vi "SVFA Power Spectral Density (1 Ch).vi"(0 "scaled signal [EU]":waveform(dbl), 2 "window":T8=1 items=["None"=0, "Hanning"=1, "Hamming"=2, "Blackman-Harris"=3, "Exact Blackman"=4, "Blackman"=5, "Flat Top"=6, "4 Term B-Harris "=7, "7 Term B-Harris"=8, "Low Sidelobe"=9, "Force"=64, "Exponential"=65, "Blackman Nuttall"=11, "Triangle"=30, "Bartlett-Hanning"=31, "Bohman"=32, "Parzen"=33, "Welch"=34, "Kaiser"=60, "Dolph-Chebyshev"=61, "Gaussian"=62], 4 "dB On (F)":bool, 5 "error in (no error)":errorcluster, 6 "desired units":enum16{"EU^2 / Hz", "EU / sqrt(Hz)"}(ring), 7 "averaging parameters":T7={"averaging mode"=enum."No averaging", "weighting mode"=enum."Exponential", "number of averages"=10, "linear mode"=enum."One shot"} {"number of averages" min=1 step=1}, 9 "restart averaging (F)":bool) -> (11 "averaging done":bool, 13 "averages completed":dbl, 14 "power spectral density [EU^2 rms / Hz]":cluster{"f0":dbl, "df":dbl, "magnitude":dbl[]}={"f0"=nan, "df"=inf, "magnitude"=[]} {"magnitude" format="%.2p"; "df" format="%.2p"; "f0" format="%.2p"}, 15 "unit label":string, 18 "spectrum info":T1={"channel name"="", "description"="", "x-axis units"=0, "spectral info"={"spectrum type"=enum."Power [Magnitude^2]", "linear/dB"=enum."linear", "window"=0, "window size"=0, "FFT size"=0}, "engineering units"=0, "custom label"="", "dB reference [EU]"=0.0, "peak units"=enum."rms", "weighting filter"=0, "spectral density?"=FALSE, "unit label"="", "spectrum skewed?"=FALSE, "complimentary spectrum units"=enum."none"} {"x-axis units" items=["Time (s)"=0, "Frequency-CB (Hz)"=1, "Frequency-CPB (Hz)"=1248, "Frequency-Arbitrary (Hz)"=2357, "Quefrency (s)"=2, "Revolutions (rev)"=3, "Order"=4, "Speed (RPM)"=11, "Speed (rad/s)"=21, "Index"=65535]; "weighting filter" items=["Linear", "A-weighting", "B-weighting", "C-weighting", "ITU-R 468-4", "Dolby", "CCITT", "C-message", "Wb", "Wc", "Wd", "We", "Wf", "Wh", "Wj", "Wk", "Wm", "AES17 20 kHz lowpass", "AES17 40 kHz lowpass", "AES17 20 kHz highpass", "AES17 40 kHz highpass"]; "dB reference [EU]" format="%.2f"; "engineering units" items=["custom..."=0, "V"=1, "A"=21, "C"=30, "pC"=31, "s"=32, "-"=29, "Pa"=2, "N"=20, "g"=3, "m/s^2"=4, "m/s"=5, "m"=6, "mm/s"=12, "mm"=13, "micron/s"=14, "micron"=15, "in/s^2"=7, "in/s"=8, "in"=9, "mil/s"=10, "mil"=11, "rad/s^2"=16, "rad/s"=17, "rad"=18, "deg/s^2"=26, "deg/s"=27, "deg"=28, "RPM"=22, "cycle/s^2"=23, "Hz"=24, "cycle"=25, "strain"=19]; "spectral info"."window" items=["None "=0, "Hanning"=1, "Hamming"=2, "Blackman-Harris"=3, "Exact Blackman"=4, "Blackman"=5, "Flat Top"=6, "4 Term B-Harris "=7, "7 Term B-Harris"=8, "Low Sidelobe"=9, "Force - Exponential"=10, "Gaussian"=62]}, 19 "error out":errorcluster)   [LabVIEW 2017]
doc: "Computes the power spectral density of <B>scaled signal [EU]</B> and returns the result in the selected units. Use the power spectral density to make repeatable measurements of the noise floor that are independent of the block size. Wire data to the <B>scaled signal [EU]</B> input to determine the polymorphic instance to use or manually select the instance."
uses:
  <vilib>/addons/_NISVFA/_Shared subVIs/Controls/svc_Window.ctl
  <vilib>/addons/_NISVFA/_Shared subVIs/Controls/svc_Spectrum Info.ctl
  <vilib>/addons/_NISVFA/_Shared subVIs/Controls/svc_X-Axis Units.ctl
  <vilib>/addons/_NISVFA/_Shared subVIs/Controls/svc_Spectrum Type.ctl
  <vilib>/addons/_NISVFA/_Shared subVIs/Controls/svc_Engineering Units Text Ring.ctl
  <vilib>/addons/_NISVFA/_Shared subVIs/Controls/svc_Weighting Filter Text Ring.ctl
  <vilib>/addons/_NISVFA/_Shared subVIs/Controls/svc_Complimentary Spectrum Units.ctl
  <vilib>/Analysis/2dsp.llb/Power Spectrum (DBL).vi
  <vilib>/Analysis/2dsp.llb/Real FFT.vi
  <vilib>/addons/_NISVFA/_Shared subVIs/Windowing/svfa_Scaled Time Domain Window (Array).vi
  <vilib>/addons/_NISVFA/_Shared subVIs/Common/svc_Get SV Channel Info.vi
  <vilib>/addons/_NISVFA/_Shared subVIs/Spectrum Averaging/svfa_No Average Array (complex).vi
  <vilib>/addons/_NISVFA/_Shared subVIs/Spectrum Averaging/svfa_Average Array (complex).vi
  <vilib>/addons/_NISVFA/_Spectrum Processing/subVIs/svfa_Peak to RMS to Peak2Peak.vi
  <vilib>/addons/_NISVFA/_Spectrum Processing/subVIs/svfa_Mag to Mag2.vi
  <vilib>/addons/_NISVFA/_Spectrum Processing/subVIs/svfa_Linear to dB.vi
  <vilib>/addons/_NISVFA/_Spectrum Processing/subVIs/svfa_dBrefA to dBrefB.vi
  <vilib>/addons/_NISVFA/_Spectrum Processing/subVIs/svfa_Spectrum to Spectral Density.vi
  <vilib>/Analysis/4window.llb/Force Window.vi
  <vilib>/Analysis/4window.llb/Force Window (DBL).vi
  <vilib>/Analysis/4window.llb/Exponential Window.vi
  <vilib>/Analysis/4window.llb/Exponential Window (DBL).vi
  <vilib>/addons/_NISVFA/_Shared subVIs/Common/svc_Get Weighting Enum and Labels.vi
  <vilib>/addons/_NISVFA/_Shared subVIs/Common/svc_Unit Label Lexical Class.vi
  <vilib>/addons/_NISVFA/_Shared subVIs/Common/svc_Engineering Units to Unit Label.vi
  <vilib>/addons/_NISVFA/_Shared subVIs/Common/svc_Format Value (DBL).vi
  <vilib>/addons/_NISVFA/_Shared subVIs/Common/svc_Window Parameters.vi
  <vilib>/Utility/error.llb/Error Cluster From Error Code.vi
  <vilib>/Analysis/0measdsp.llb/Scaled Time Domain Window.vi
  <vilib>/Analysis/0measdsp.llb/Scaled Time Domain Window (DBL).vi
  <vilib>/addons/_NISVFA/_Spectrum Processing/subVIs/svfa_Spectrum Info Window to windowTd Type Def.vi
  <vilib>/addons/_NISVFA/_Shared subVIs/Common/svc_Get Window Info.vi
  <vilib>/addons/_NISVFA/_Shared subVIs/Common/svc_Channel Info to Spectrum Info.vi
  <vilib>/addons/_NISVFA/_Shared subVIs/Common/svc_Unit Label to Engineering Units.vi
  <vilib>/Analysis/NI_AALPro.lvlib
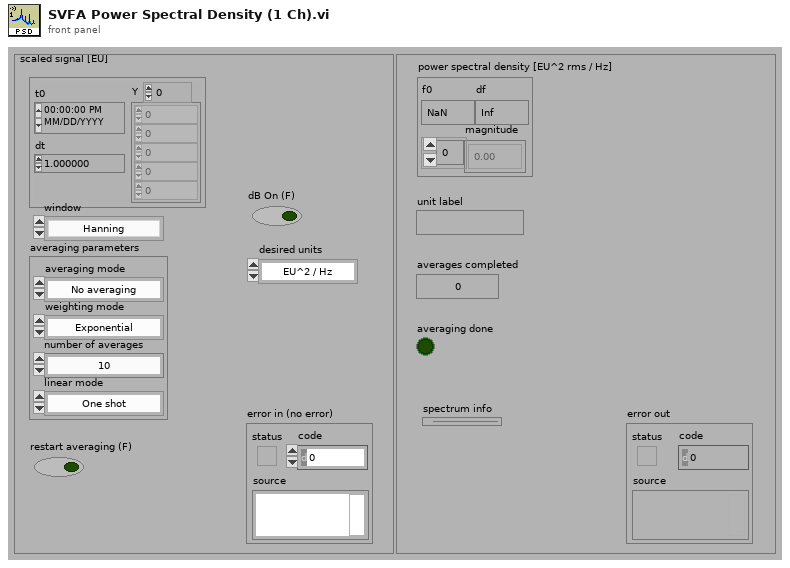
[diagram p1: front panel]
types:
  T1 = typedef "svc_Spectrum Info.ctl" = cluster{"channel name":string, "description":string, "x-axis units":T2, "spectral info":cluster{"spectrum type":T3, "linear/dB":enum16{"linear", "dB"}, "window":u16, "window size":i32, "FFT size":i32}, "engineering units":T4, "custom label":string, "dB reference [EU]":dbl, "peak units":enum16{"rms", "peak", "peak-peak"}, "weighting filter":T5, "spectral density?":bool, "unit label":string, "spectrum skewed?":bool, "complimentary spectrum units":T6}
  T2 = typedef "svc_X-Axis Units.ctl" = u16
  T3 = typedef "svc_Spectrum Type.ctl" = enum16{"FFT Spectrum [complex]", "Amplitude [Magnitude]", "Power [Magnitude^2]", "Cross Spectrum [complex]", "Frequency Response [Complex]"}
  T4 = typedef "svc_Engineering Units Text Ring.ctl" = u16
  T5 = typedef "svc_Weighting Filter Text Ring.ctl" = u16
  T6 = typedef "svc_Complimentary Spectrum Units.ctl" = enum16{"none", "radians", "degrees", "cycles", "imaginary"}
  T7 = cluster{"averaging mode":enum16{"No averaging", "Vector averaging", "RMS averaging", "Peak hold"}, "weighting mode":enum16{"Linear", "Exponential"}, "number of averages":u32, "linear mode":enum16{"One shot", "Auto restart"}}
  T8 = typedef "svc_Window.ctl" = u32
  T9 = cluster{"linear/dB":enum16{"no change", "linear", "dB"}, "dB reference (0: no change)":dbl, "power/magnitude":enum16{"no change", "power", "magnitude"}, "view":enum16{"no change", "rms", "peak", "peak-peak"}}
  T10 = enum16{"Restart processing", "Continue processing", "Skip processing"}
  T11 = enum16{"no change", "spectrum", "spectral density"}
  T12 = enum16{"No averaging", "Vector averaging", "RMS averaging", "Peak hold"}
  T13 = cluster{"complex FFT":cdb[], "real FFT":dbl[], "f0":dbl, "df":dbl, "averages completed":dbl, "averaging parameters":cluster{"averaging mode":enum16{"No averaging", "Vector averaging", "RMS averaging", "Peak hold"}, "weighting mode":enum16{"Linear", "Exponential"}, "number of averages":u32, "linear mode":enum16{"One shot", "Auto restart"}}}
  T14 = cluster{"complex FFT":cdb[], "Mag/Real FFT":dbl[], "f0":dbl, "df":dbl, "averages completed":dbl, "averaging parameters":cluster{"averaging mode":enum16{"No averaging", "Vector averaging", "RMS averaging", "Peak hold"}, "weighting mode":enum16{"Linear", "Exponential"}, "number of averages":u32, "linear mode":enum16{"One shot", "Auto restart"}}}
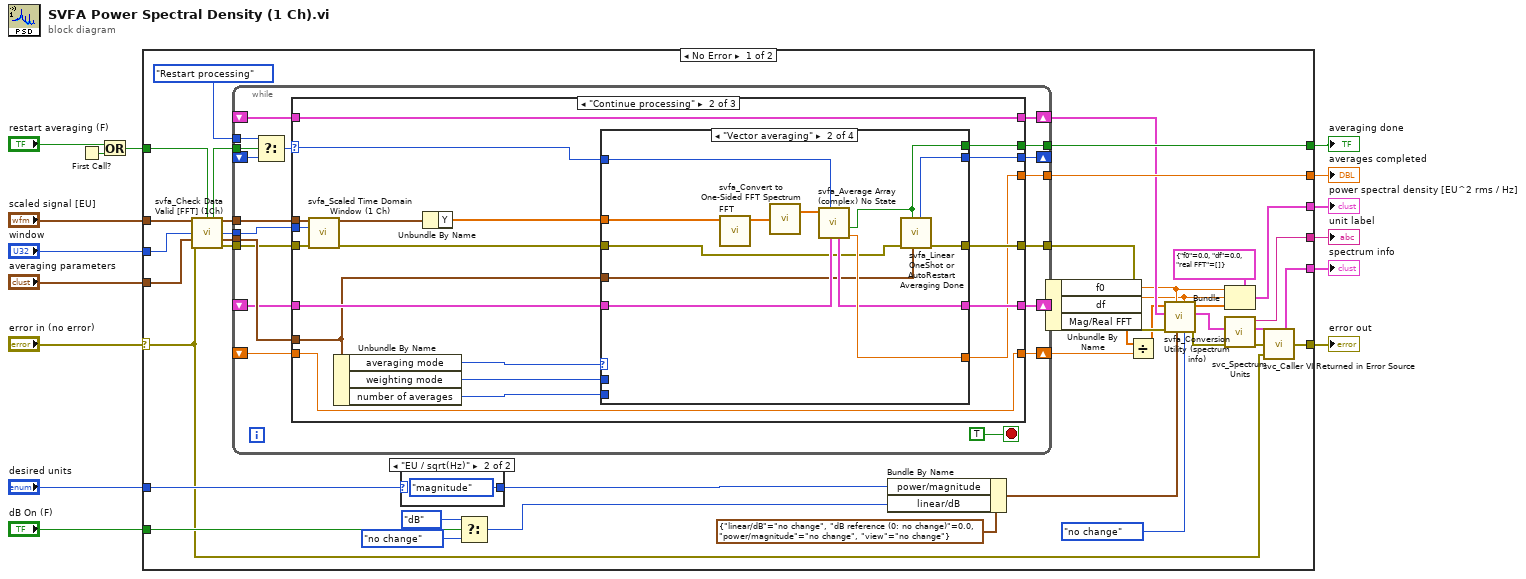
[diagram p0: block diagram]
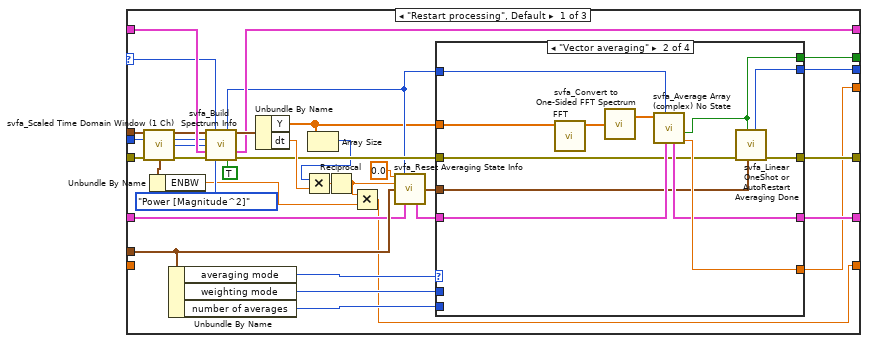
[diagram p2: hidden frame]
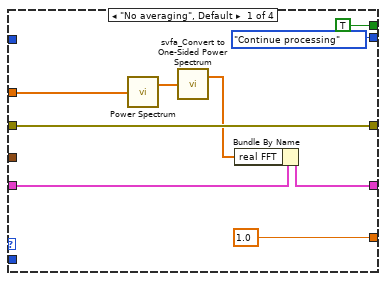
[diagram p3: hidden frame]
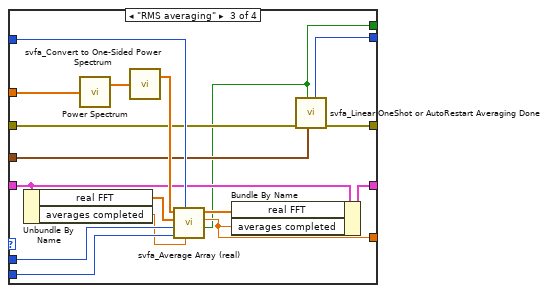
[diagram p4: hidden frame]
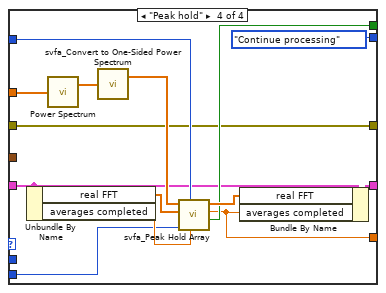
[diagram p5: hidden frame]
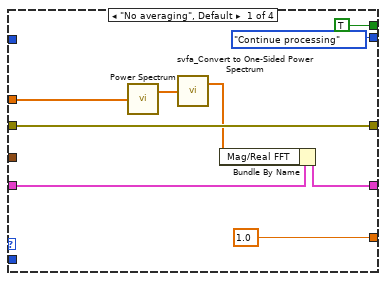
[diagram p6: hidden frame]
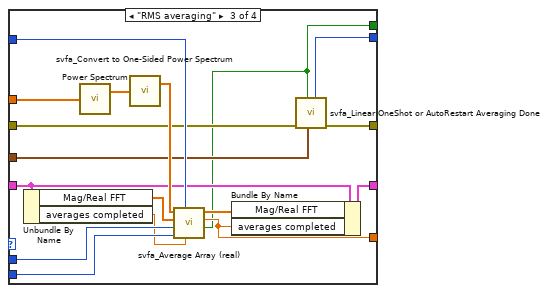
[diagram p7: hidden frame]
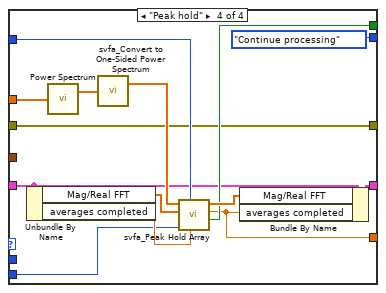
[diagram p8: hidden frame]
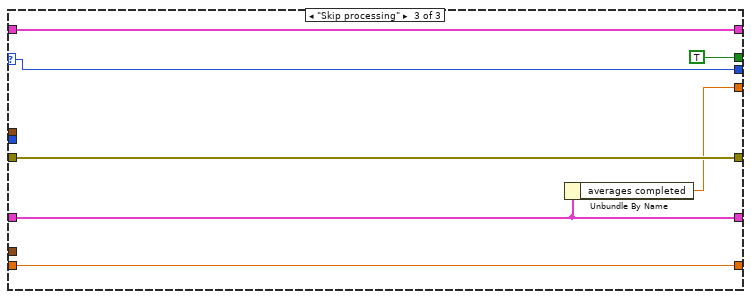
[diagram p9: hidden frame]
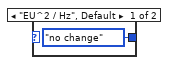
[diagram p10: hidden frame]
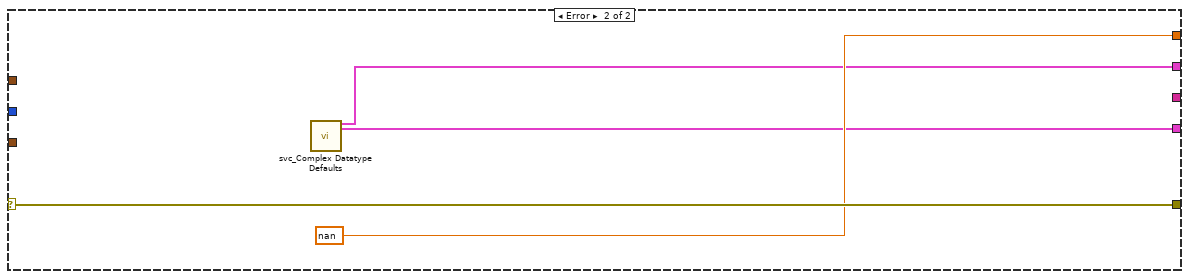
[diagram p11: hidden frame]
diagram:
  n1 = First Call?() -> (First Call?: T/F=w5:bool)
  n2 = Or(x="restart averaging (F)", y=w5) -> (x .or. y?=w3:bool)
  n3 = case shown="No Error" "error in (no error)" {
    selector: "error in (no error)" -> [w42 w245]
    tunnel: "scaled signal [EU]" -> [w54 _]
    tunnel: w3 -> [w51 _]
    tunnel: [w49 w245] -> w14
    tunnel: "averaging parameters" -> [w52 _]
    tunnel: "window" -> [w53 _]
    tunnel: [w20 w243] -> w10
    tunnel: "dB On (F)" -> [w50 _]
    tunnel: [w33 nan ("averages completed")] -> w8
    tunnel: [w32 _] -> w7
    tunnel: [w22 w242] -> w6
    tunnel: "desired units" -> [w48 _]
    tunnel: [w19 _] -> w1
    frame No Error {
      n4 = call <vilib>:"svfa_Check Data Valid [FFT] (1Ch).vi"("signal in [X]"=w54, "restart averaging (F)"=w51, "window"=w53, "averaging parameters"=w52, "error in (no error)"=w42) -> ("restart averaging"=w38:bool, "dup signal in [X]"=w36:waveform(dbl), "dup window"=w34:T8, "dup averaging parameters"=w35:T7, "error out"=w37:errorcluster)  [unwired: 6 in]
      n5 = while {
        tunnel: w34 -> [w66]
        shift-left: _ -> [w67]
        shift-right: [w59] -> w40
        tunnel: [w71] -> w33
        tunnel: [w72] -> w32
        tunnel: [w57] -> w25
        tunnel: w35 -> [w73]
        tunnel: w37 -> [w69]
        tunnel: w36 -> [w70]
        shift-right: [w58] -> w26
        shift-left: _ -> [w65]
        shift-right: [w64] -> _
        shift-left: _ -> [w62]
        tunnel: w38 -> [w63]
        tunnel: T10."Restart processing" ("t") -> [w60]
        shift-right: [w56] -> w17
        shift-left: _ -> [w55]
        stop <- TRUE stop-if-true
        n6 = Select(t=w60, s=w63, f=w62) -> (s? t:f=w61:T10)
        n7 = case shown="\"Continue processing\"" w61 {
          selector: w61 -> [w107 w164 w237]
          tunnel: w73 -> [w92 w162 _]
          tunnel: [w88 w175 w238] -> w57
          tunnel: [w82 w172 TRUE ("averaging done?")] -> w72
          tunnel: [w81 w171 w234] -> w71
          tunnel: w70 -> [w105 w180 _]
          tunnel: w69 -> [w103 w178 w238]
          tunnel: [w89 w176 w237] -> w64
          tunnel: [w87 w174 w235] -> w59
          tunnel: w67 -> [w91 w167 w235]
          tunnel: w66 -> [w104 w179 _]
          tunnel: [w99 w165 w236] -> w58
          tunnel: w65 -> [w109 w165 w236]
          tunnel: [w78 w163 w233] -> w56
          tunnel: w55 -> [_ w163 w233]
          frame "Restart processing", Default {
            n8 = call <vilib>:"svfa_Scaled Time Domain Window (1 Ch).vi"("Signal in [X]"=w105, "window"=w104, "error in"=w103) -> ("Windowed Waveform"=w100:waveform(dbl), "dup window"=w101:T8, "window length"=w94:i32, "window constants"=w97:cluster{"ENBW":dbl, "CG":dbl}, "error out"=w102:errorcluster)  [unwired: 7 in, 1 out]
            n9 = Unbundle By Name(w97) -> ("ENBW"=w96:dbl)
            n10 = Unbundle By Name(w92) -> ("averaging mode"=w83:T12, "weighting mode"=w80:enum16{"Linear", "Exponential"}, "number of averages"=w79:u32)
            n11 = call <vilib>:"svfa_Build Spectrum Info.vi"("scaled signal [EU]"=w100, "processing control"=w107, "window"=w101, "window size"=w94, "spectrum info in"=w109, "error in (no error)"=w102, "spectrum type"=svc_Spectrum_Type."Power [Magnitude^2]", "spectral density?"=TRUE) -> ("dup processing control"=w84:T10, "dup scaled signal [EU]"=w106:waveform(dbl), "spectrum info out"=w99:T1, "error out"=w90:errorcluster)  [unwired: 4 in]
            n12 = Unbundle By Name ("Get Waveform Components")(w106) -> ("Y"=w77:dbl[], "dt"=w95:dbl)
            n13 = Array Size(array=w77) -> (size(s)=w76:i32)
            n14 = Multiply(x=w76, y=w95) -> (x*y=w75:dbl)
            n15 = Reciprocal(x=w75) -> (1/x=w74:dbl)
            n16 = Multiply(x=w74, y=w96) -> (x*y=w78:dbl)
            n17 = call <vilib>:"svfa_Reset Averaging State Info.vi"("f0"=0.0, "processing control"=w84, "df"=w74, "averaging parameters"=w92, "averaging state info in"=w91) -> ("dup averaging parameters"=w85:T7, "averaging state info out"=w86:T13)  [unwired: 9 in]
            n18 = case shown="\"Vector averaging\"" w83 {
              tunnel: [w115 w121 w133 w149] -> w88
              tunnel: [1.0 ("averages completed") w129 w137 w152] -> w81
              tunnel: [TRUE ("averaging done") w119 w131 w153] -> w82
              tunnel: w90 -> [w115 w120 w134 w149]
              tunnel: w85 -> [_ w123 w135 _]
              tunnel: w84 -> [_ w130 w140 w158]
              tunnel: w77 -> [w116 w127 w146 w160]
              tunnel: [w110 w124 w141 w151] -> w87
              tunnel: w86 -> [w111 w128 w139 w150]
              tunnel: w80 -> [_ _ w145 _]
              tunnel: w79 -> [_ _ w144 w155]
              tunnel: [T10."Continue processing" ("processing control") w122 w132 T10."Continue processing" ("processing control")] -> w89
              frame "No averaging", Default {
                n19 = call-poly <vilib>:"Power Spectrum.vi"("X"=w116) -> ("Power Spectrum"=w117:dbl[])  [unwired: 1 out]
                n20 = call <vilib>:"svfa_Convert to One-Sided Power Spectrum.vi"("two-sided power spectrum"=w117) -> ("one-sided power spectrum"=w112:dbl[])  [unwired: 1 out]
                n21 = Bundle By Name(cluster=w111, "real FFT"=w112) -> (w110:T13)
              }
              frame "Vector averaging" {
                n22 = call-poly <vilib>:"FFT.vi"("X"=w127) -> ("FFT {X}"=w126:cdb[])  [unwired: 9 in, 1 out]
                n23 = call <vilib>:"svfa_Convert to One-Sided FFT Spectrum.vi"("two-sided FFT spectrum"=w126) -> ("one-sided FFT spectrum"=w125:cdb[])  [unwired: 1 out]
                n24 = call <vilib>:"svfa_Average Array (complex) No State.vi"("averaging state info in"=w128, "processing control"=w130, "array"=w125) -> ("averages completed"=w129:dbl, "averaging done"=w119:bool, "averaging state info out"=w124:T14)  [unwired: 5 in, 1 out]
                n25 = call <vilib>:"svfa_Linear OneShot or AutoRestart Averaging Done.vi"("averaging parameters"=w123, "averaging done"=w119, "error in (no error)"=w120) -> ("error out"=w121:errorcluster, "processing control"=w122:T10)  [unwired: 7 in]
              }
              frame "RMS averaging" {
                n26 = Unbundle By Name(w139) -> ("real FFT"=w142:dbl[], "averages completed"=w138:dbl)
                n27 = call-poly <vilib>:"Power Spectrum.vi"("X"=w146) -> ("Power Spectrum"=w147:dbl[])  [unwired: 1 out]
                n28 = call <vilib>:"svfa_Convert to One-Sided Power Spectrum.vi"("two-sided power spectrum"=w147) -> ("one-sided power spectrum"=w143:dbl[])  [unwired: 1 out]
                n29 = call <vilib>:"svfa_Average Array (real).vi"("averages completed in"=w138, "processing control"=w140, "number of averages"=w144, "weighting mode"=w145, "previous average array"=w142, "array"=w143) -> ("averaging done"=w131:bool, "averages completed out"=w137:dbl, "average array"=w136:dbl[])  [unwired: 3 in]
                n30 = Bundle By Name(cluster=w139, "real FFT"=w136, "averages completed"=w137) -> (w141:T13)
                n31 = call <vilib>:"svfa_Linear OneShot or AutoRestart Averaging Done.vi"("averaging parameters"=w135, "averaging done"=w131, "error in (no error)"=w134) -> ("error out"=w133:errorcluster, "processing control"=w132:T10)  [unwired: 7 in]
              }
              frame "Peak hold" {
                n32 = Unbundle By Name(w150) -> ("real FFT"=w157:dbl[], "averages completed"=w156:dbl)
                n33 = call-poly <vilib>:"Power Spectrum.vi"("X"=w160) -> ("Power Spectrum"=w161:dbl[])  [unwired: 1 out]
                n34 = call <vilib>:"svfa_Convert to One-Sided Power Spectrum.vi"("two-sided power spectrum"=w161) -> ("one-sided power spectrum"=w159:dbl[])  [unwired: 1 out]
                n35 = call <vilib>:"svfa_Peak Hold Array.vi"("averages completed in"=w156, "processing control"=w158, "number of averages"=w155, "previous peak array"=w157, "array"=w159) -> ("averaging done"=w153:bool, "averages completed out"=w152:dbl, "peak array"=w154:dbl[])  [unwired: 4 in]
                n36 = Bundle By Name(cluster=w150, "real FFT"=w154, "averages completed"=w152) -> (w151:T13)
              }
            }
          }
          frame "Continue processing" {
            n37 = call <vilib>:"svfa_Scaled Time Domain Window (1 Ch).vi"("Signal in [X]"=w180, "window"=w179, "error in"=w178) -> ("Windowed Waveform"=w168:waveform(dbl), "error out"=w166:errorcluster)  [unwired: 7 in, 4 out]
            n38 = Unbundle By Name(w162) -> ("averaging mode"=w173:T12, "weighting mode"=w170:enum16{"Linear", "Exponential"}, "number of averages"=w169:u32)
            n39 = Unbundle By Name ("Get Waveform Components")(w168) -> ("Y"=w177:dbl[])
            n40 = case shown="\"Vector averaging\"" w173 {
              tunnel: [w186 w192 w204 w220] -> w175
              tunnel: [1.0 ("averages completed") w200 w208 w223] -> w171
              tunnel: [TRUE ("averaging done") w190 w202 w224] -> w172
              tunnel: w166 -> [w186 w191 w205 w220]
              tunnel: w162 -> [_ w194 w206 _]
              tunnel: w164 -> [_ w201 w211 w229]
              tunnel: w177 -> [w187 w198 w217 w231]
              tunnel: [w181 w195 w212 w222] -> w174
              tunnel: w167 -> [w182 w199 w210 w221]
              tunnel: w170 -> [_ _ w216 _]
              tunnel: w169 -> [_ _ w215 w226]
              tunnel: [T10."Continue processing" ("processing control") w193 w203 T10."Continue processing" ("processing control")] -> w176
              frame "No averaging", Default {
                n41 = call-poly <vilib>:"Power Spectrum.vi"("X"=w187) -> ("Power Spectrum"=w188:dbl[])  [unwired: 1 out]
                n42 = call <vilib>:"svfa_Convert to One-Sided Power Spectrum.vi"("two-sided power spectrum"=w188) -> ("one-sided power spectrum"=w183:dbl[])  [unwired: 1 out]
                n43 = Bundle By Name(cluster=w182, "Mag/Real FFT"=w183) -> (w181:T14)
              }
              frame "Vector averaging" {
                n44 = call-poly <vilib>:"FFT.vi"("X"=w198) -> ("FFT {X}"=w197:cdb[])  [unwired: 9 in, 1 out]
                n45 = call <vilib>:"svfa_Convert to One-Sided FFT Spectrum.vi"("two-sided FFT spectrum"=w197) -> ("one-sided FFT spectrum"=w196:cdb[])  [unwired: 1 out]
                n46 = call <vilib>:"svfa_Average Array (complex) No State.vi"("averaging state info in"=w199, "processing control"=w201, "array"=w196) -> ("averages completed"=w200:dbl, "averaging done"=w190:bool, "averaging state info out"=w195:T14)  [unwired: 5 in, 1 out]
                n47 = call <vilib>:"svfa_Linear OneShot or AutoRestart Averaging Done.vi"("averaging parameters"=w194, "averaging done"=w190, "error in (no error)"=w191) -> ("error out"=w192:errorcluster, "processing control"=w193:T10)  [unwired: 7 in]
              }
              frame "RMS averaging" {
                n48 = Unbundle By Name(w210) -> ("Mag/Real FFT"=w213:dbl[], "averages completed"=w209:dbl)
                n49 = call-poly <vilib>:"Power Spectrum.vi"("X"=w217) -> ("Power Spectrum"=w218:dbl[])  [unwired: 1 out]
                n50 = call <vilib>:"svfa_Convert to One-Sided Power Spectrum.vi"("two-sided power spectrum"=w218) -> ("one-sided power spectrum"=w214:dbl[])  [unwired: 1 out]
                n51 = call <vilib>:"svfa_Average Array (real).vi"("averages completed in"=w209, "processing control"=w211, "number of averages"=w215, "weighting mode"=w216, "previous average array"=w213, "array"=w214) -> ("averaging done"=w202:bool, "averages completed out"=w208:dbl, "average array"=w207:dbl[])  [unwired: 3 in]
                n52 = Bundle By Name(cluster=w210, "Mag/Real FFT"=w207, "averages completed"=w208) -> (w212:T14)
                n53 = call <vilib>:"svfa_Linear OneShot or AutoRestart Averaging Done.vi"("averaging parameters"=w206, "averaging done"=w202, "error in (no error)"=w205) -> ("error out"=w204:errorcluster, "processing control"=w203:T10)  [unwired: 7 in]
              }
              frame "Peak hold" {
                n54 = Unbundle By Name(w221) -> ("Mag/Real FFT"=w228:dbl[], "averages completed"=w227:dbl)
                n55 = call-poly <vilib>:"Power Spectrum.vi"("X"=w231) -> ("Power Spectrum"=w232:dbl[])  [unwired: 1 out]
                n56 = call <vilib>:"svfa_Convert to One-Sided Power Spectrum.vi"("two-sided power spectrum"=w232) -> ("one-sided power spectrum"=w230:dbl[])  [unwired: 1 out]
                n57 = call <vilib>:"svfa_Peak Hold Array.vi"("averages completed in"=w227, "processing control"=w229, "number of averages"=w226, "previous peak array"=w228, "array"=w230) -> ("averaging done"=w224:bool, "averages completed out"=w223:dbl, "peak array"=w225:dbl[])  [unwired: 4 in]
                n58 = Bundle By Name(cluster=w221, "Mag/Real FFT"=w225, "averages completed"=w223) -> (w222:T14)
              }
            }
          }
          frame "Skip processing" {
            n59 = Unbundle By Name(w235) -> ("averages completed"=w234:dbl)
          }
        }
      }
      n60 = case shown="\"EU / sqrt(Hz)\"" w48 {
        tunnel: [enum16{"no change", "power", "magnitude"}."no change" ("power/magnitude") enum16{"no change", "power", "magnitude"}."magnitude" ("power/magnitude")] -> w47
        frame "EU^2 / Hz", Default {
        }
        frame "EU / sqrt(Hz)" {
        }
      }
      n61 = Select(t=enum16{"no change", "linear", "dB"}."dB" ("linear/dB"), s=w50, f=enum16{"no change", "linear", "dB"}."no change" ("linear/dB")) -> (s? t:f=w44:enum16{"no change", "linear", "dB"})
      n62 = Bundle By Name(cluster=T9 {"linear/dB"=enum."no change", "dB reference (0: no change)"=0.0, "power/magnitude"=enum."no change", "view"=enum."no change"} ("desired scaling"), "power/magnitude"=w47, "linear/dB"=w44) -> (w28:T9)
      n63 = Unbundle By Name(w40) -> ("f0"=w24:dbl, "df"=w23:dbl, "Mag/Real FFT"=w16:dbl[])
      n64 = Divide(x=w16, y=w17) -> (x/y=w18:dbl[])
      n65 = call <vilib>:"svfa_Conversion Utility (spectrum info).vi"("spectral density desired"=T11."no change", "dx"=w23, "desired scaling"=w28, "x0"=w24, "error in (no error)"=w25, "spectrum info in"=w26, "input signal"=w18) -> ("error out"=w31:errorcluster, "spectrum info out"=w30:T1, "converted signal"=w29:dbl[])  [unwired: 2 in]
      n66 = Bundle(cluster=cluster{"f0":dbl, "df":dbl, "real FFT":dbl[]} {"f0"=0.0, "df"=0.0, "real FFT"=[]}, "f0"=w24, "df"=w23, "real FFT"=w29) -> (w20:cluster{"f0":dbl, "df":dbl, "real FFT":dbl[]})
      n67 = call <vilib>:"svc_Spectrum Units.vi"("error in (no error)"=w31, "spectrum info in"=w30) -> ("error out"=w21:errorcluster, "spectrum info out"=w22:T1, "unit label"=w19:string)  [unwired: 2 in, 1 out]
      n68 = call <vilib>:"svc_Caller VI Returned in Error Source.vi"("warning input to caller"=w42, "error in (no error)"=w21) -> ("error out"=w49:errorcluster)  [unwired: 3 in]
    }
    frame Error {
      n69 = call <vilib>:"svc_Complex Datatype Defaults.vi"() -> ("empty spectrum"=w243:cluster{"f0":dbl, "df":dbl, "magnitude":dbl[]}, "dead spectrum info"=w242:T1)  [unwired: 11 in, 7 out]
    }
  }
  "error out" <- w14
  "power spectral density [EU^2 rms / Hz]" <- w10
  "unit label" <- w1
  "averaging done" <- w7
  "averages completed" <- w8
  "spectrum info" <- w6
